vi "Get Image Data and Que.vi"(6 "Acquisition count":i32, 8 "error in (no error)":errorcluster, 9 "Exp params":T2 {"TSFrames" min=1 step=1; "TSfps" min=0.001 max=90.0 step=0.001 format="%_4g"}, 10 "Refnum in":T3, 11 "Queue in":refnum<queue>) -> (1 "Logging Cluster":T1={"Image Data Array"=[], "Buffer Number"=0, "Timestamp (um)"=0, "Exp params"={"Experiment Type"="Dynamic Time Series", "Experiment Name"="Experiment_1", "ExpPath"=path "D:/Data", "Save As"="TIFF", "TSFrames"=1000, "TSfps"=1.0, "Streaming"=FALSE, "tdms ref"=refnum, "frame #"=0, "Full Path"=path "", "PeakOnQueue"=FALSE}} {"Exp params"."TSFrames" min=1 step=1; "Exp params"."TSfps" min=0.001 max=90.0 step=0.001 format="%_4g"}, 2 "Session Out":T3, 3 "Queue out":refnum<queue>)   [LabVIEW 2020]
uses:
  _controls/Logging Cluster.ctl
  _controls/Exp Params.ctl
  <vilib>/userDefined/High Color/IMAQdx.ctl
  <vilib>/vision/driver/IMAQdx.llb/IMAQdx Buffer Number Mode.ctl
  _controls/Timer_actions.ctl
  <vilib>/vision/driver/NI_Vision_Acquisition_Software.lvlib
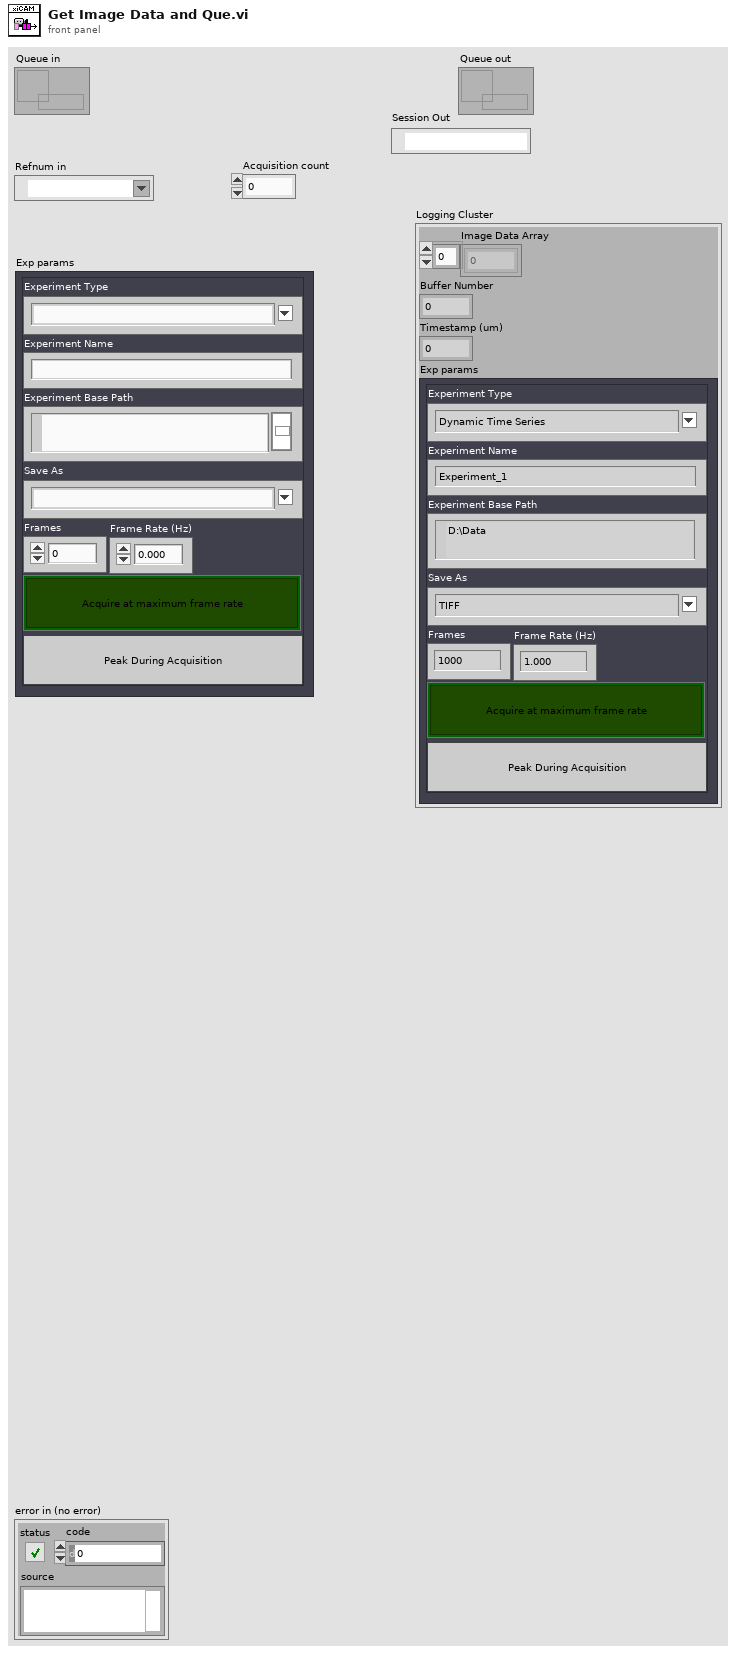
[diagram p1: front panel]
types:
  T1 = typedef "Logging Cluster.ctl" = cluster{"Image Data Array":u8[], "Buffer Number":i32, "Timestamp (um)":u64, "Exp params":T2}
  T2 = typedef "Exp Params.ctl" = cluster{"Experiment Type":string, "Experiment Name":string, "ExpPath":path, "Save As":string, "TSFrames":i32, "TSfps":dbl, "Streaming":bool, "tdms ref":refnum<k34>, "frame #":i64, "Full Path":path, "PeakOnQueue":bool}
  T3 = typedef "IMAQdx.ctl" = refnum<k21>
  T4 = typedef "Timer_actions.ctl" = enum16{"Reset", "Snap", "Total"}
  T5 = typedef "NI_Vision_Acquisition_Software.lvlib/IMAQdx Buffer Number Mode.ctl" = enum32{"Next", "Last", "Buffer Number", "Every", "Last New"}
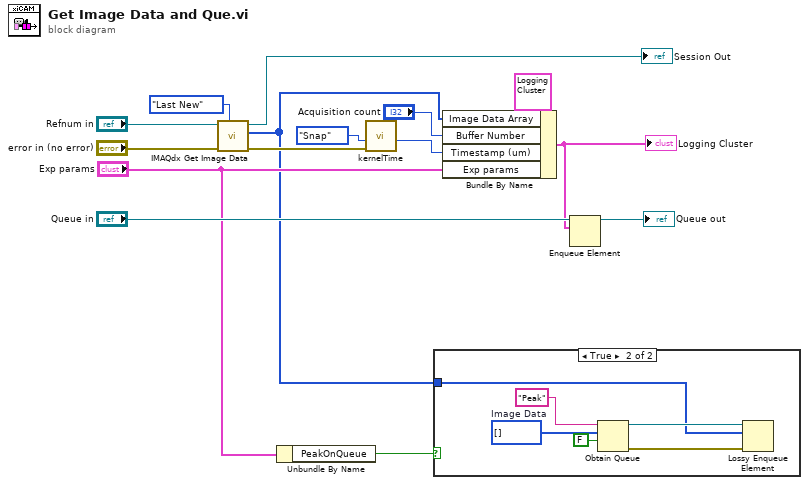
[diagram p0: block diagram]
diagram:
  n1 = call <vilib>:"IMAQdx Get Image Data.vi"("Buffer Number Mode (Next)"=IMAQdx_Buffer_Number_Mode."Last New", "error in"="error in (no error)", "Session In"="Refnum in") -> ("error out"=w12:errorcluster, "Image Data Array"=w1:u8[], "Session Out"=→"Session Out":T3)  [unwired: 5 in, 1 out]
  n2 = Unbundle By Name("Exp params") -> ("PeakOnQueue"=w2:bool)
  n3 = call "kernelTime.vi"("error in (no error) in"=w12, "Action (Snap)"=Timer_actions."Snap") -> ("Microseconds"=w6:u64)  [unwired: 8 in, 1 out]
  n4 = case shown="True" w2 {
    tunnel: w1 -> [_ w16]
    frame False {
    }
    frame True {
      w21 = u8[] []  # Image Data
      n5 = Obtain Queue(name (unnamed)="Peak", element data type=w21, create if not found? (T)=FALSE) -> (queue out=w19:refnum<queue>, error out=w17:errorcluster)  [unwired: 2 in, 1 out]
      n6 = Lossy Enqueue Element(queue=w19, element=w16, error in (no error)=w17) -> ()  [unwired: 4 out]
    }
  }
  n7 = Bundle By Name(cluster=T1 {"Image Data Array"=[], "Buffer Number"=0, "Timestamp (um)"=0, "Exp params"={"Experiment Type"="", "Experiment Name"="", "ExpPath"=path "", "Save As"="", "TSFrames"=0, "TSfps"=0.0, "Streaming"=FALSE, "tdms ref"=refnum, "frame #"=0, "Full Path"=path "", "PeakOnQueue"=FALSE}} ("Logging Cluster"), "Image Data Array"=w1, "Buffer Number"="Acquisition count", "Timestamp (um)"=w6, "Exp params"="Exp params") -> (w4:T1)
  "Logging Cluster" <- w4
  n8 = Enqueue Element(queue="Queue in", element=w4) -> (queue out=→"Queue out":refnum<queue>)  [unwired: 2 in, 2 out]
